vi "Table_Globals.vi"() -> ()   [LabVIEW 2012, in "TableSupportLib.lvlib"]
uses:
  TableSupportLib.lvlib
panel:
  in  "Limits Header":string="Name,Path,High,High Warning,Low Warning,Low"
  in  "Template":string="Template"
  in  "Path":string="Path"
  in  "Limits":string="Limits"
  in  "Invalid Tag":string="INVALID: "
  in  "Data_Value Column":i32=1
  in  "Data_Path Column":i32=4
  in  "NumericConversion":string="%.2p"
  in  "Exit":string="Exit"
  in  "Init":string="Init"
  in  "Name Column":i32
  in  "OK":string="OK"
  in  "Path Column":i32=1
  in  "Remove":string="Remove"
  in  "Add":string="Add"
  in  "QueueName":string="SelectChannels"
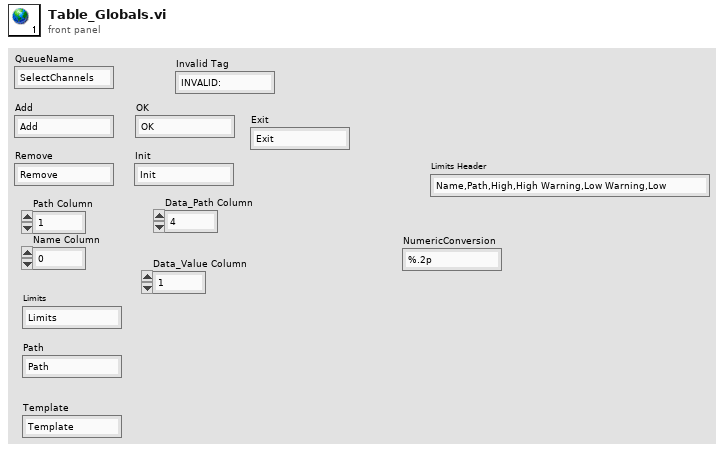
[diagram p1: front panel]
diagram:
